vi "Set TC Reference.vi"(7 "Reference Source (T: Internal)":bool=TRUE, 8 "error in (no error)":errorcluster, 9 "Temperature Units (22: Temperature in degrees Celsius)":u32(ring)=22 items=["Unitless", "Frequency in units of hertz", "Frequency in units of kilohertz", "Frequency in units of megahertz", "Volts in units of microvolts", "Volts in units of millivolts", "Volts in units of volts", "Volts in units of kilovolts", "Current in units of microamperes", "Current in units of milliamps", "Current in units of amps", "Percent", "Parts-per-million", "Volts in units of decibels referenced to 1 milliwatt into 600 W load", "Resistance in units of ohms", "Resistance in units of kilohms", "Resistance in units of megohms", "Capacitance in units of nanofarads", "Capacitance in units of picofarads", "Capacitance in units of  microfarads", "Capacitance in units of millifarads", "Capacitance in units of farads", "Temperature in degrees Celsius", "Temperature in degrees Fahrenheit", "Period in units of nanoseconds", "Period in units of microseconds", "Period in units of milliseconds", "Period in units of seconds", "Pound-force pre square inch", "Meters of mercury", "Inches of mercury", "Inches of water", "Feet of water", "Meters of water", "Bar", "Pascal", "Grams per centimeter squared", "Inches of water @ 60 degrees Farhenheit", "Decibels"], 10 "External Reference Value (0.0)":dbl format="%.3f", 11 "VISA resource name":refnum<visa-resource-name>) -> (0 "error out":errorcluster, 3 "VISA resource name out":refnum<visa-resource-name>)   [LabVIEW 2011, in "Fluke 5XXX Series Multicalibrators.lvlib"]
doc: "This VI sets whether the internal temperature sensor (INT) or an external reference value (EXT) is used for Thermocouple (TC) outputs and measurements.\n\nIf the INT is selected, value to use as the reference for the thermocouple reference junction temperature is ignored.\n\nOnce set, the Calibrator retains reference setting until power off or reset.\n\nNote:\n\nThis VI is available only for instrument models 5500A and 5520A."
uses:
  Fluke 5XXX Series Multicalibrators.lvlib
panel:
  # "Internal"
  # "External"
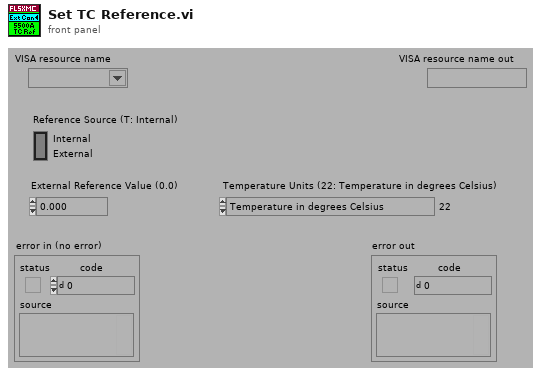
[diagram p1: front panel]
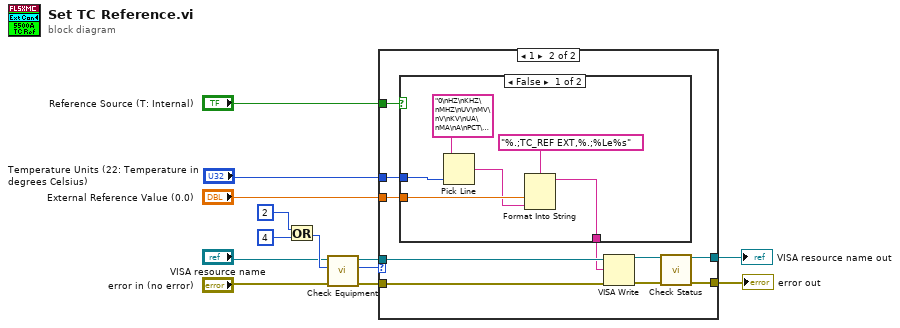
[diagram p0: block diagram]
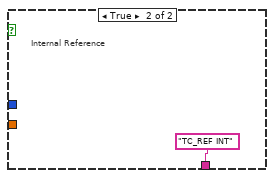
[diagram p3: hidden frame]
diagram:
  n1 = Or(x=2 ("Numeric"), y=4 ("Numeric")) -> (x .or. y?=w8:i32)
  n2 = call "Check Equipment.vi"("error in (no error)"="error in (no error)", "Bit Mask"=w8, "VISA resource name"="VISA resource name") -> ("error out"=w13:errorcluster, "Present?"=w12:u32, "VISA resource name out"=w11:refnum<visa-resource-name>)  [unwired: 6 in]
  n3 = case shown="1" w12 {
    tunnel: "Temperature Units (22: Temperature in degrees Celsius)" -> [_ w19]
    tunnel: [w14 w22] -> w2
    tunnel: w13 -> [w15 w25]
    tunnel: w11 -> [w14 w24]
    tunnel: [w15 w23] -> w3
    tunnel: "Reference Source (T: Internal)" -> [_ w18]
    tunnel: "External Reference Value (0.0)" -> [_ w17]
    frame 0, Default {
    }
    frame 1 {
      n4 = case shown="False" w18 {
        tunnel: w19 -> [w30 _]
        tunnel: w17 -> [w29 _]
        tunnel: [w26 "TC_REF INT"] -> w16
        frame False {
          n5 = Pick Line(multi-line string="0\nHZ\nKHZ\nMHZ\nUV\nMV\nV\nKV\nUA\nMA\nA\nPCT\nPPM\nDBM\nOHM\nKOHM\nMOHM\nNF\nPF\nUF\nMF\nF\nCEL\nFAR\nNS\nUS\nMS\nS\nPSI\nMHG\nINHG\nINH2O\nFTH2O\nMH2O\nBAR\nPAL\nG/CM2\nINH2O60F\nDB", line index=w30) -> (output string=w27:string)  [unwired: 1 in]
          n6 = Format Into String(format string="%.;TC_REF EXT,%.;%Le%s" ("Reset Command"), w29, w27) -> (resulting string=w26:string)  [unwired: 2 in, 1 out]
        }
        frame True {
          # "Internal Reference"
        }
      }
      n7 = VISA Write(VISA resource name=w24, write buffer=w16, error in (no error)=w25) -> (VISA resource name out=w21:refnum<visa-resource-name>, error out=w20:errorcluster)  [unwired: 1 out]
      n8 = call "Check Status.vi"("VISA resource name"=w21, "error in (no error)"=w20) -> ("VISA resource name out"=w22:refnum<visa-resource-name>, "error out"=w23:errorcluster)  [unwired: 12 in]
    }
  }
  "VISA resource name out" <- w2
  "error out" <- w3
